vi "S706 Warnings.vi"(8 "Fehler (Eingang, kein Fehler)":errorcluster) -> (0 "error out":errorcluster, 3 "SWE":bool)   [LabVIEW 2014]
uses:
  <vilib>/CANopenLib/CANOPEN.llb/CANopen SDO Create.vi
  <vilib>/CANopenLib/CANOPEN.llb/CANopen SDO Read [U32].vi
  <vilib>/CANopenLib/CANOPEN.llb/CANopen SDO Close.vi
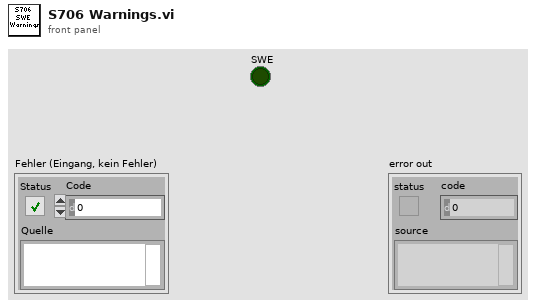
[diagram p1: front panel]
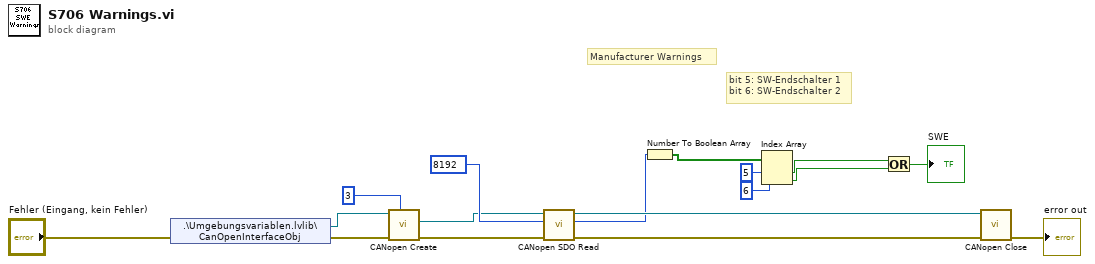
[diagram p0: block diagram]
diagram:
  # "Manufacturer Warnings"
  # "bit 5: SW-Endschalter 1\nbit 6: SW-Endschalter 2"
  n1 = shared-variable ".\\Umgebungsvariablen.lvlib\\CanOpenInterfaceObj"(error in="Fehler (Eingang, kein Fehler)") -> (w16:refnum<k20>, error out=w17:errorcluster)
  n2 = call-poly <vilib>:"CANopen Create.vi"("node-ID"=u8 3, "error in (no error)"=w17, "interface object in"=w16) -> ("error out"=w12:errorcluster, "SDO object out"=w13:refnum<k20>)  [unwired: 6 in, 1 out]
  n3 = call-poly <vilib>:"CANopen SDO Read.vi"("error in (no error)"=w12, "object index"=u16 8192, "SDO object in"=w13) -> ("error out"=w8:errorcluster, "U32 data"=w7:u32, "SDO object out"=w9:refnum<k20>)  [unwired: 5 in, 1 out]
  n4 = Number To Boolean Array(number=w7) -> (Boolean array=w6:bool[])
  n5 = Index Array(array=w6, index #1=5 ("Index"), index #2=6 ("Index")) -> (element #1=w3:bool, element #2=w2:bool)
  n6 = Or(x=w3, y=w2) -> (x .or. y?=→"SWE":bool)
  n7 = call-poly <vilib>:"CANopen Close.vi"("error in (no error)"=w8, "SDO object in"=w9) -> ("error out"=→"error out":errorcluster)  [unwired: 9 in]
